vi "Configure Digital Pattern Output Trigger.vi"(8 "error in (no error)":errorcluster, 9 "Trigger Slope (Positive)":bool=TRUE, 10 "Trigger Enable (No)":bool, 11 "VISA resource name":refnum<visa-resource-name>) -> (0 "error out":errorcluster, 3 "VISA resource name out":refnum<visa-resource-name>)   [LabVIEW 2017, in "Keithley 3390.lvlib"]
doc: "Configures the Digital Pattern Output Trigger"
uses:
  Keithley 3390.lvlib
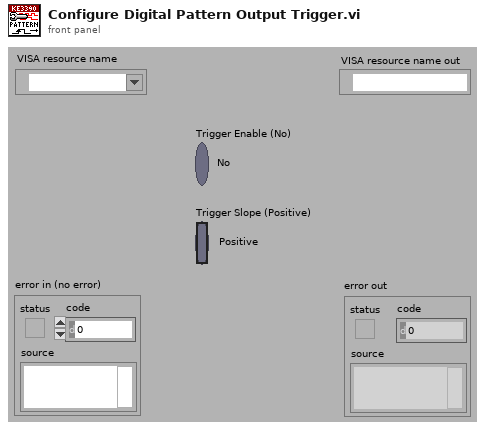
[diagram p1: front panel]
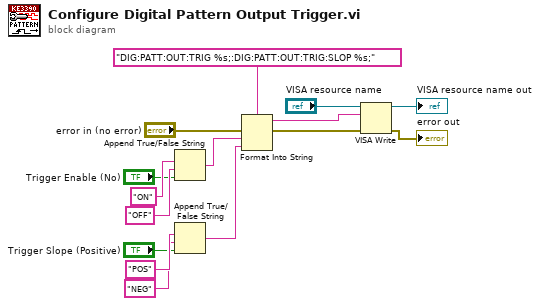
[diagram p0: block diagram]
diagram:
  n1 = Append True/False String(1:"Trigger Enable (No)", 2:"OFF" ("false string"), 3:"ON" ("true string")) -> (0:w3:string)  [unwired: 1 in]
  n2 = Append True/False String(1:"Trigger Slope (Positive)", 2:"NEG" ("false string"), 3:"POS" ("true string")) -> (0:w4:string)  [unwired: 1 in]
  n3 = Format Into String(format string="DIG:PATT:OUT:TRIG %s;:DIG:PATT:OUT:TRIG:SLOP %s;", error in="error in (no error)", w3, w4) -> (resulting string=w1:string, error out=w2:errorcluster)  [unwired: 1 in]
  n4 = VISA Write(VISA resource name="VISA resource name", write buffer=w1, error in (no error)=w2) -> (VISA resource name out=→"VISA resource name out":refnum<visa-resource-name>, error out=→"error out":errorcluster)  [unwired: 1 out]
